vi "Lock Automation Reference.vi"(8 "error in":errorcluster, 10 "Sequence Context":T1, 11 "Launcher in":refnum<class "Launcher.lvclass">) -> (0 "error out":errorcluster, 3 "Launcher out":refnum<class "Launcher.lvclass">)   [LabVIEW 2019, in "Launcher.lvlib" / "Launcher.lvclass"]
uses:
  Library/Launcher.lvclass
  <vilib>/addons/TestStand/_TSLegacy.llb/LabVIEW Test - Sequence Context.ctl
  Library/Launcher.lvclass/Launcher.ctl
  builds/Base Software/Base Software.lvlibp/Base Software Messages/Update Automation Reference Msg/Update Automation Reference Msg.lvclass
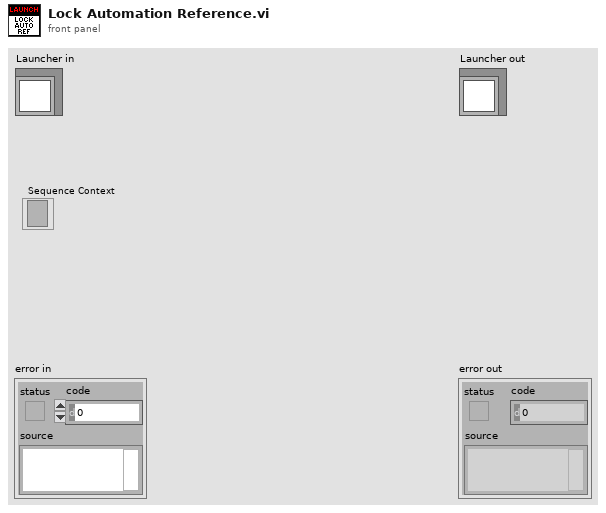
[diagram p1: front panel]
types:
  T1 = typedef "LabVIEW Test - Sequence Context.ctl" = refnum<k7>
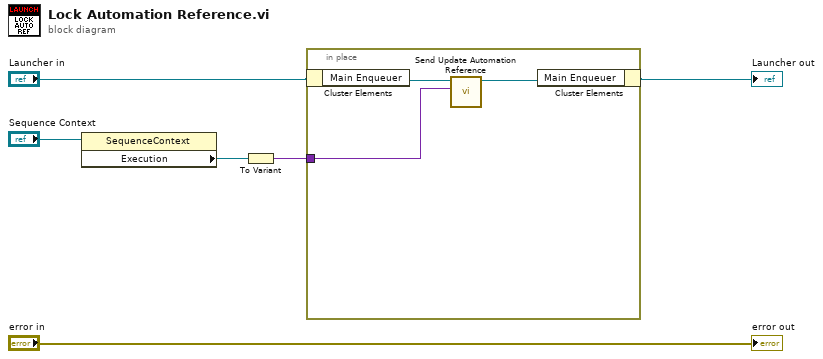
[diagram p0: block diagram]
diagram:
  n1 = property class="SequenceContext"(reference="Sequence Context") -> ("Execution"=w5:refnum<k7>)  [unwired: 1 in, 2 out]
  n2 = To Variant(anything=w5) -> (Variant=w2:variant)
  n3 = in-place {
    in-place-border: w2 -> [w7]
    n4 = in-place-cluster #1("Launcher in") -> ("Main Enqueuer"=w9:refnum<class "Message Enqueuer.lvclass">)
    n5 = call "Send Update Automation Reference.vi"("Automation"=w7, "Message Enqueuer"=w9) -> ("Message Enqueuer out"=w8:refnum<class "Message Enqueuer.lvclass">)  [unwired: 8 in, 1 out]
    n6 = in-place-cluster #1("Main Enqueuer"=w8) -> (→"Launcher out":refnum<class "Launcher.lvclass">)
  }
  "error out" <- "error in"
